vi "GetStringsAndValues.vi"(8 "error in":errorcluster, 11 "Ring in":refnum<class "Ring.lvclass">) -> (0 "error out":errorcluster, 3 "Ring out":refnum<class "Ring.lvclass">)   [LabVIEW 2014, in "Raspberry Pi Compatible Compiler for LabVIEW.lvlib" / "Ring.lvclass"]
uses:
  Ring.lvclass
  Ring.lvclass/Ring.ctl
  <vilib>/Utility/VariantDataType/VariantType.lvlib
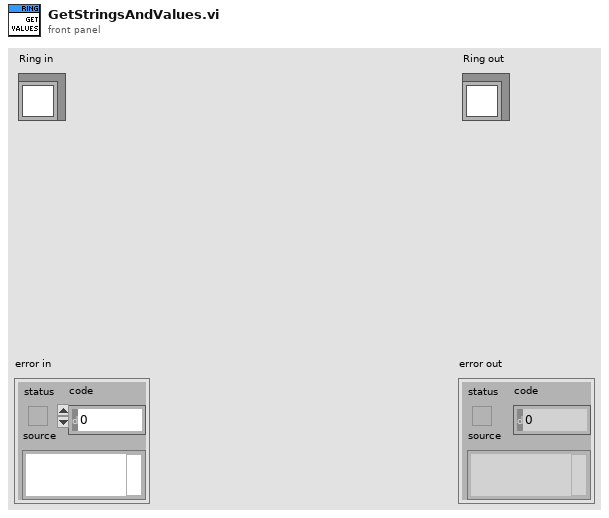
[diagram p1: front panel]
types:
  T1 = typedef "LVStringsAndValuesArrayTypeDef.ctl" = cluster{"String":string, "Value":ext}[]
  T2 = typedef "LVNumericRepresentation.ctl" = enum32{"Extended Precision", "Double Precision", "Single Precision", "Long", "Word", "Byte", "Unsigned Long", "Unsigned Word", "Unsigned Byte", "Complex Extended", "Complex Double", "Complex Single", "Quad", "Unsigned Quad", "Fixed-Point"}
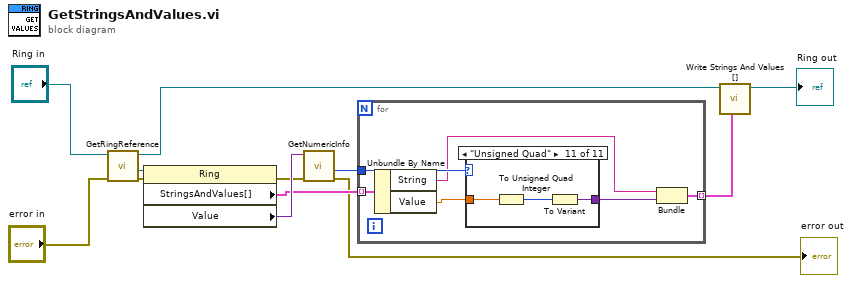
[diagram p0: block diagram]
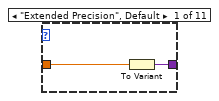
[diagram p2: hidden frame]
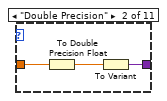
[diagram p3: hidden frame]
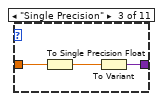
[diagram p4: hidden frame]
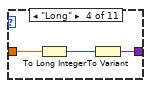
[diagram p5: hidden frame]
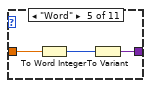
[diagram p6: hidden frame]
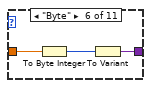
[diagram p7: hidden frame]
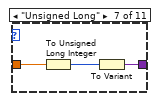
[diagram p8: hidden frame]
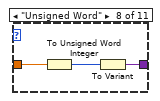
[diagram p9: hidden frame]
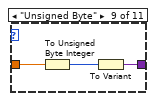
[diagram p10: hidden frame]
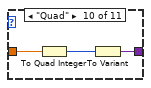
[diagram p11: hidden frame]
diagram:
  n1 = call "GetRingReference.vi"("error in"="error in", "Ring in"="Ring in") -> ("error out"=w7:errorcluster, "Ring reference"=w6:refnum<vi>, "Ring out"=w3:refnum<class "Ring.lvclass">)  [unwired: 7 in]
  n2 = property class="Ring"(reference=w6, error in=w7) -> (error out=w5:errorcluster, "StringsAndValues[]"=w8:T1, "Value"=w9:variant)  [unwired: 1 out]
  n3 = call <vilib>:"GetNumericInfo.vi"("error in (no error)"=w5, "Variant"=w9) -> ("error out"=→"error out":errorcluster, "representation"=w10:T2)  [unwired: 6 in, 2 out]
  n4 = for {
    tunnel: w8 -> [w18] mode=indexing
    tunnel: w10 -> [w17]
    tunnel: [w13] -> w1 mode=indexing
    n5 = Unbundle By Name(w18) -> ("String"=w14:string, "Value"=w16:ext)
    n6 = case shown="\"Unsigned Quad\"" w17 {
      tunnel: w16 -> [w20 w23 w26 w29 w32 w35 w38 w41 w44 w47 w50]
      tunnel: [w19 w22 w25 w28 w31 w34 w37 w40 w43 w46 w49] -> w15
      frame "Extended Precision", Default {
        n7 = To Variant(anything=w20) -> (Variant=w19:variant)
      }
      frame "Double Precision" {
        n8 = To Double Precision Float(number=w23) -> (double precision float=w21:dbl)
        n9 = To Variant(anything=w21) -> (Variant=w22:variant)
      }
      frame "Single Precision" {
        n10 = To Single Precision Float(number=w26) -> (single precision float=w24:sgl)
        n11 = To Variant(anything=w24) -> (Variant=w25:variant)
      }
      frame "Long" {
        n12 = To Long Integer(number=w29) -> (32bit integer=w27:i32)
        n13 = To Variant(anything=w27) -> (Variant=w28:variant)
      }
      frame "Word" {
        n14 = To Word Integer(number=w32) -> (16bit integer=w30:i16)
        n15 = To Variant(anything=w30) -> (Variant=w31:variant)
      }
      frame "Byte" {
        n16 = To Byte Integer(number=w35) -> (8bit integer=w33:i8)
        n17 = To Variant(anything=w33) -> (Variant=w34:variant)
      }
      frame "Unsigned Long" {
        n18 = To Unsigned Long Integer(number=w38) -> (unsigned 32bit integer=w36:u32)
        n19 = To Variant(anything=w36) -> (Variant=w37:variant)
      }
      frame "Unsigned Word" {
        n20 = To Unsigned Word Integer(number=w41) -> (unsigned 16bit integer=w39:u16)
        n21 = To Variant(anything=w39) -> (Variant=w40:variant)
      }
      frame "Unsigned Byte" {
        n22 = To Unsigned Byte Integer(number=w44) -> (unsigned 8bit integer=w42:u8)
        n23 = To Variant(anything=w42) -> (Variant=w43:variant)
      }
      frame "Quad" {
        n24 = To Quad Integer(1:w47) -> (0:w45:i64)
        n25 = To Variant(anything=w45) -> (Variant=w46:variant)
      }
      frame "Unsigned Quad" {
        n26 = To Unsigned Quad Integer(1:w50) -> (0:w48:u64)
        n27 = To Variant(anything=w48) -> (Variant=w49:variant)
      }
    }
    n28 = Bundle("String"=w14, "Variant"=w15) -> (w13:cluster{"String":string, "Variant":variant})  [unwired: 1 in]
  }
  n29 = call "Write Strings And Values [].vi"("Strings And Values []"=w1, "Ring in"=w3) -> ("Ring out"=→"Ring out":refnum<class "Ring.lvclass">)  [unwired: 7 in]
